vi "_write.vi"(8 "Error in (no error)":errorcluster, 10 "Log in":T1 {"Priority" items=["EMERGENCY", "ALERT", "CRITICAL", "ERROR", "WARNING", "NOTICE", "INFO", "DEBUG"]}, 11 "LogWriterDb in":refnum<class "LogWriterDb.lvclass">) -> (0 "Error out":errorcluster, 3 "LogWriterDb out":refnum<class "LogWriterDb.lvclass">)   [LabVIEW 2011, in "LogWriterDb.lvclass"]
uses:
  LogWriterDb.lvclass
  Log/LogCluster.ctl
  Log/PrioritiesRing.ctl
  LogWriterDb.lvclass/LogWriterDb.ctl
  <vilib>/addons/database/NI_Database_API.lvlib
  Log/Log.lvclass
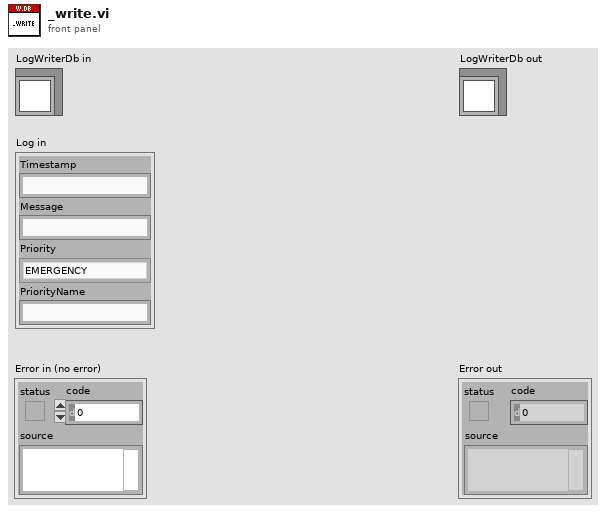
[diagram p1: front panel]
types:
  T1 = typedef "Log.lvclass/LogCluster.ctl" = cluster{"Timestamp":string, "Message":string, "Priority":T2, "PriorityName":string}
  T2 = typedef "Log.lvclass/PrioritiesRing.ctl" = u32
  T3 = typedef "NI_Database_API.lvlib/Conn ObjectReference.ctl" = refnum<k1>
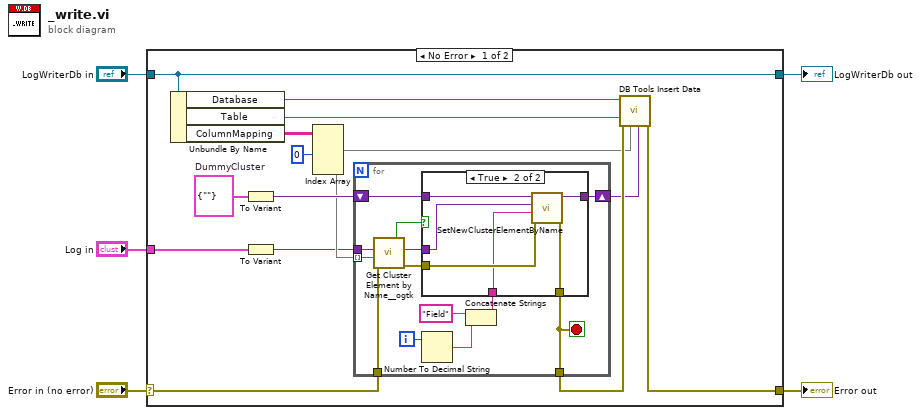
[diagram p0: block diagram]
diagram:
  n1 = case shown="No Error" "Error in (no error)" {
    selector: "Error in (no error)" -> [w16 w43]
    tunnel: [w17 w43] -> w4
    tunnel: [w20 w42] -> w2
    tunnel: "LogWriterDb in" -> [w20 w42]
    tunnel: "Log in" -> [w7 _]
    frame No Error {
      w13 = cluster{"Field0":string} {"Field0"=""}  # DummyCluster
      n2 = Unbundle By Name(w20) -> ("Database"=w19:T3, "Table"=w18:string, "ColumnMapping"=w11:string[][])
      n3 = To Variant(anything=w13) -> (Variant=w12:variant)
      n4 = To Variant(anything=w7) -> (Variant=w6:variant)
      n5 = Index Array(array=w11, index (col) #1=0 ("disabled index (col)")) -> (element #1=w9:string[], element #2=w10:string[])  [unwired: 3 in]
      n6 = for {
        tunnel: w6 -> [w33]
        tunnel: w10 -> [w25] mode=indexing
        shift-right: [w31] -> w14
        shift-left: w12 -> [w32]
        tunnel: [w27] -> w15
        tunnel: w16 -> [w28]
        i -> [w24]
        stop <- w27 stop-if-true
        n7 = call <userlib>:"Get Cluster Element by Name__ogtk.vi"("error in (no error)"=w28, "Element Name"=w25, "Cluster"=w33) -> ("error out"=w29:errorcluster, "found?"=w26:bool, "VElement"=w30:variant)  [unwired: 6 in]
        n8 = Number To Decimal String(number=w24) -> (decimal integer string=w21:string)  [unwired: 1 in]
        n9 = Concatenate Strings("Field", w21) -> (w23:string)
        n10 = case shown="True" w26 {
          tunnel: w32 -> [w35 w41]
          tunnel: [w35 w40] -> w31
          tunnel: w30 -> [_ w39]
          tunnel: w29 -> [w34 w38]
          tunnel: [w34 w37] -> w27
          tunnel: w23 -> [_ w36]
          frame False {
          }
          frame True {
            n11 = call "SetNewClusterElementByName.vi"("error in (no error)"=w38, "Element Name (\"\": New Element Data Name)"=w36, "New Element Value"=w39, "Cluster"=w41) -> ("error out"=w37:errorcluster, "VCluster out"=w40:variant)  [unwired: 6 in]
          }
        }
      }
      n12 = call <vilib>:"DB Tools Insert Data.vi"("data"=w14, "error in (no error)"=w15, "columns"=w9, "table"=w18, "connection reference"=w19) -> ("error out"=w17:errorcluster)  [unwired: 5 in, 1 out]
    }
    frame Error {
    }
  }
  "Error out" <- w4
  "LogWriterDb out" <- w2
